vi "Lab Panel V4.91.vi"() -> ()   [LabVIEW 2013] (continued)
                          tunnel: w4008 -> [_ _]
                          tunnel: w4007 -> [_ w4049]
                          tunnel: w4006 -> [_ w4048]
                          tunnel: w4005 -> [_ w4013]
                          tunnel: w4002 -> [_ w4045]
                          tunnel: w4001 -> [_ w4044]
                          tunnel: w4000 -> [_ w4042]
                          tunnel: w3999 -> [_ w4034]
                          frame False {
                          }
                          frame True {
                            n2185 = local read "TDMS LAB02-2"() -> (w4047:refnum<k34>)
                            n2186 = Build Array(w4044) -> (w4039:dbl[])
                            n2187 = Build Array(w4042) -> (w4038:dbl[])
                            n2188 = Build Array(w4049) -> (w4037:dbl[])
                            n2189 = Build Array(w4050) -> (w4036:dbl[])
                            n2190 = Build Array(w4045) -> (w4041:dbl[])
                            n2191 = Build Array(w4043) -> (w4040:dbl[])
                            n2192 = Build Array(w4048) -> (w4035:dbl[])
                            n2193 = Build Array("AMPS ON", "AMPS OFF", "VOLTS", "PF", "TEMP Live", "TEMP Neut", "CYCLE") -> (w4018:string[])
                            n2194 = Bundle By Name("Y"=w4041, "t0"=w4034) -> (w4033:waveform(dbl))  [unwired: 1 in]
                            n2195 = Bundle By Name("Y"=w4040, "t0"=w4034) -> (w4032:waveform(dbl))  [unwired: 1 in]
                            n2196 = Bundle By Name("Y"=w4039, "t0"=w4034) -> (w4031:waveform(dbl))  [unwired: 1 in]
                            n2197 = Bundle By Name("Y"=w4038, "t0"=w4034) -> (w4030:waveform(dbl))  [unwired: 1 in]
                            n2198 = Bundle By Name("Y"=w4037, "t0"=w4034) -> (w4029:waveform(dbl))  [unwired: 1 in]
                            n2199 = Bundle By Name("Y"=w4036, "t0"=w4034) -> (w4028:waveform(dbl))  [unwired: 1 in]
                            n2200 = Bundle By Name("Y"=w4035, "t0"=w4034) -> (w4027:waveform(dbl))  [unwired: 1 in]
                            n2201 = Build Array(w4033, w4032, w4031, w4030, w4029, w4028, w4027) -> (w4026:waveform(dbl)[])
                            n2202 = TDMS Write(0:w4047, 5:"TEST VALUES", 7:w4018, 9:w4026) -> (4:w4017:refnum<k34>, 6:w4016:string, 15:w4015:errorcluster)  [unwired: 2 in, 1 out]
                            n2203 = TDMS Write(0:w4017, 5:w4016, 7:"TIME", 9:w4013, 11:w4015) -> (15:w4012:errorcluster)  [unwired: 1 in, 3 out]
                            n2204 = local write "data file error"(w4012) -> ()
                          }
                        }
                      }
                    }
                  }
                }
              }
              frame #4 {
                n2205 = case shown="True" w4051 {
                  tunnel: w4055 -> [_ w4060]
                  tunnel: w4054 -> [_ w4059]
                  tunnel: w4053 -> [_ w4057]
                  tunnel: w4052 -> [_ w4056]
                  frame False {
                  }
                  frame True {
                    n2206 = local read "DISP LAB03-1"() -> (w4061:T4)
                    n2207 = local read "SIG LAB03-1"() -> (w4062:T2)
                    n2208 = local read "ON L03-1"() -> (w4058:cluster{"amps":dbl, "volts":dbl, "pf":dbl})
                    n2209 = Unbundle(w4062) -> ("AMPS"=w4068:dbl, "VOLTS"=w4066:dbl, "PF"=w4065:dbl, "Tmp Live"=w4064:dbl, "Tmp Neut"=w4067:dbl)
                    n2210 = Unbundle(w4061) -> ("CYCLE"=w4063:dbl)  [unwired: 2 out]
                    n2211 = stacked-sequence {
                      tunnel: w4068 -> [w4072 w4091]
                      tunnel: w4067 -> [_ w4090]
                      tunnel: w4066 -> [w4071 w4089]
                      tunnel: w4065 -> [w4070 w4088]
                      tunnel: w4064 -> [_ w4087]
                      tunnel: w4063 -> [_ w4086]
                      tunnel: w4060 -> [_ w4085]
                      tunnel: w4059 -> [w4073 _]
                      tunnel: w4058 -> [w4069 w4083]
                      tunnel: w4057 -> [_ w4084]
                      tunnel: w4056 -> [_ w4079]
                      frame #0 {
                        n2212 = case shown="True" w4073 {
                          tunnel: w4072 -> [_ w4078]
                          tunnel: w4071 -> [_ w4077]
                          tunnel: w4070 -> [_ w4076]
                          tunnel: w4069 -> [_ w4074]
                          frame False {
                          }
                          frame True {
                            n2213 = Bundle(cluster=w4074, "amps"=w4078, "volts"=w4077, "pf"=w4076) -> (w4075:cluster{"amps":dbl, "volts":dbl, "pf":dbl})
                            n2214 = local write "ON L03-1"(w4075) -> ()
                          }
                        }
                      }
                      frame #1 {
                        n2215 = Unbundle(w4083) -> ("amps"=w4082:dbl, "volts"=w4081:dbl, "pf"=w4080:dbl)
                        n2216 = case shown="True" w4084 {
                          tunnel: w4091 -> [_ w4123]
                          tunnel: w4090 -> [_ w4130]
                          tunnel: w4089 -> [_ _]
                          tunnel: w4088 -> [_ _]
                          tunnel: w4087 -> [_ w4129]
                          tunnel: w4086 -> [_ w4128]
                          tunnel: w4085 -> [_ w4093]
                          tunnel: w4082 -> [_ w4125]
                          tunnel: w4081 -> [_ w4124]
                          tunnel: w4080 -> [_ w4122]
                          tunnel: w4079 -> [_ w4114]
                          frame False {
                          }
                          frame True {
                            n2217 = local read "TDMS LAB03-1"() -> (w4127:refnum<k34>)
                            n2218 = Build Array(w4124) -> (w4119:dbl[])
                            n2219 = Build Array(w4122) -> (w4118:dbl[])
                            n2220 = Build Array(w4129) -> (w4117:dbl[])
                            n2221 = Build Array(w4130) -> (w4116:dbl[])
                            n2222 = Build Array(w4125) -> (w4121:dbl[])
                            n2223 = Build Array(w4123) -> (w4120:dbl[])
                            n2224 = Build Array(w4128) -> (w4115:dbl[])
                            n2225 = Build Array("AMPS ON", "AMPS OFF", "VOLTS", "PF", "TEMP Live", "TEMP Neut", "CYCLE") -> (w4098:string[])
                            n2226 = Bundle By Name("Y"=w4121, "t0"=w4114) -> (w4113:waveform(dbl))  [unwired: 1 in]
                            n2227 = Bundle By Name("Y"=w4120, "t0"=w4114) -> (w4112:waveform(dbl))  [unwired: 1 in]
                            n2228 = Bundle By Name("Y"=w4119, "t0"=w4114) -> (w4111:waveform(dbl))  [unwired: 1 in]
                            n2229 = Bundle By Name("Y"=w4118, "t0"=w4114) -> (w4110:waveform(dbl))  [unwired: 1 in]
                            n2230 = Bundle By Name("Y"=w4117, "t0"=w4114) -> (w4109:waveform(dbl))  [unwired: 1 in]
                            n2231 = Bundle By Name("Y"=w4116, "t0"=w4114) -> (w4108:waveform(dbl))  [unwired: 1 in]
                            n2232 = Bundle By Name("Y"=w4115, "t0"=w4114) -> (w4107:waveform(dbl))  [unwired: 1 in]
                            n2233 = Build Array(w4113, w4112, w4111, w4110, w4109, w4108, w4107) -> (w4106:waveform(dbl)[])
                            n2234 = TDMS Write(0:w4127, 5:"TEST VALUES", 7:w4098, 9:w4106) -> (4:w4097:refnum<k34>, 6:w4096:string, 15:w4095:errorcluster)  [unwired: 2 in, 1 out]
                            n2235 = TDMS Write(0:w4097, 5:w4096, 7:"TIME", 9:w4093, 11:w4095) -> (15:w4092:errorcluster)  [unwired: 1 in, 3 out]
                            n2236 = local write "data file error"(w4092) -> ()
                          }
                        }
                      }
                    }
                  }
                }
              }
              frame #5 {
                n2237 = case shown="True" w4131 {
                  tunnel: w4135 -> [_ w4140]
                  tunnel: w4134 -> [_ w4139]
                  tunnel: w4133 -> [_ w4137]
                  tunnel: w4132 -> [_ w4136]
                  frame False {
                  }
                  frame True {
                    n2238 = local read "DISP LAB03-2"() -> (w4141:T4)
                    n2239 = local read "SIG LAB03-2"() -> (w4142:T2)
                    n2240 = local read "ON L03-2"() -> (w4138:cluster{"amps":dbl, "volts":dbl, "pf":dbl})
                    n2241 = Unbundle(w4142) -> ("AMPS"=w4148:dbl, "VOLTS"=w4146:dbl, "PF"=w4145:dbl, "Tmp Live"=w4144:dbl, "Tmp Neut"=w4147:dbl)
                    n2242 = Unbundle(w4141) -> ("CYCLE"=w4143:dbl)  [unwired: 2 out]
                    n2243 = stacked-sequence {
                      tunnel: w4148 -> [w4152 w4171]
                      tunnel: w4147 -> [_ w4170]
                      tunnel: w4146 -> [w4151 w4169]
                      tunnel: w4145 -> [w4150 w4168]
                      tunnel: w4144 -> [_ w4167]
                      tunnel: w4143 -> [_ w4166]
                      tunnel: w4140 -> [_ w4165]
                      tunnel: w4139 -> [w4153 _]
                      tunnel: w4138 -> [w4149 w4163]
                      tunnel: w4137 -> [_ w4164]
                      tunnel: w4136 -> [_ w4159]
                      frame #0 {
                        n2244 = case shown="True" w4153 {
                          tunnel: w4152 -> [_ w4158]
                          tunnel: w4151 -> [_ w4157]
                          tunnel: w4150 -> [_ w4156]
                          tunnel: w4149 -> [_ w4154]
                          frame False {
                          }
                          frame True {
                            n2245 = Bundle(cluster=w4154, "amps"=w4158, "volts"=w4157, "pf"=w4156) -> (w4155:cluster{"amps":dbl, "volts":dbl, "pf":dbl})
                            n2246 = local write "ON L03-2"(w4155) -> ()
                          }
                        }
                      }
                      frame #1 {
                        n2247 = Unbundle(w4163) -> ("amps"=w4162:dbl, "volts"=w4161:dbl, "pf"=w4160:dbl)
                        n2248 = case shown="True" w4164 {
                          tunnel: w4171 -> [_ w4203]
                          tunnel: w4170 -> [_ w4210]
                          tunnel: w4169 -> [_ _]
                          tunnel: w4168 -> [_ _]
                          tunnel: w4167 -> [_ w4209]
                          tunnel: w4166 -> [_ w4208]
                          tunnel: w4165 -> [_ w4173]
                          tunnel: w4162 -> [_ w4205]
                          tunnel: w4161 -> [_ w4204]
                          tunnel: w4160 -> [_ w4202]
                          tunnel: w4159 -> [_ w4194]
                          frame False {
                          }
                          frame True {
                            n2249 = local read "TDMS LAB03-2"() -> (w4207:refnum<k34>)
                            n2250 = Build Array(w4204) -> (w4199:dbl[])
                            n2251 = Build Array(w4202) -> (w4198:dbl[])
                            n2252 = Build Array(w4209) -> (w4197:dbl[])
                            n2253 = Build Array(w4210) -> (w4196:dbl[])
                            n2254 = Build Array(w4205) -> (w4201:dbl[])
                            n2255 = Build Array(w4203) -> (w4200:dbl[])
                            n2256 = Build Array(w4208) -> (w4195:dbl[])
                            n2257 = Build Array("AMPS ON", "AMPS OFF", "VOLTS", "PF", "TEMP Live", "TEMP Neut", "CYCLE") -> (w4178:string[])
                            n2258 = Bundle By Name("Y"=w4201, "t0"=w4194) -> (w4193:waveform(dbl))  [unwired: 1 in]
                            n2259 = Bundle By Name("Y"=w4200, "t0"=w4194) -> (w4192:waveform(dbl))  [unwired: 1 in]
                            n2260 = Bundle By Name("Y"=w4199, "t0"=w4194) -> (w4191:waveform(dbl))  [unwired: 1 in]
                            n2261 = Bundle By Name("Y"=w4198, "t0"=w4194) -> (w4190:waveform(dbl))  [unwired: 1 in]
                            n2262 = Bundle By Name("Y"=w4197, "t0"=w4194) -> (w4189:waveform(dbl))  [unwired: 1 in]
                            n2263 = Bundle By Name("Y"=w4196, "t0"=w4194) -> (w4188:waveform(dbl))  [unwired: 1 in]
                            n2264 = Bundle By Name("Y"=w4195, "t0"=w4194) -> (w4187:waveform(dbl))  [unwired: 1 in]
                            n2265 = Build Array(w4193, w4192, w4191, w4190, w4189, w4188, w4187) -> (w4186:waveform(dbl)[])
                            n2266 = TDMS Write(0:w4207, 5:"TEST VALUES", 7:w4178, 9:w4186) -> (4:w4177:refnum<k34>, 6:w4176:string, 15:w4175:errorcluster)  [unwired: 2 in, 1 out]
                            n2267 = TDMS Write(0:w4177, 5:w4176, 7:"TIME", 9:w4173, 11:w4175) -> (15:w4172:errorcluster)  [unwired: 1 in, 3 out]
                            n2268 = local write "data file error"(w4172) -> ()
                          }
                        }
                      }
                    }
                  }
                }
              }
              frame #6 {
                n2269 = case shown="True" w4211 {
                  tunnel: w4215 -> [_ w4220]
                  tunnel: w4214 -> [_ w4219]
                  tunnel: w4213 -> [_ w4217]
                  tunnel: w4212 -> [_ w4216]
                  frame False {
                  }
                  frame True {
                    n2270 = local read "DISP LAB04-1"() -> (w4221:T4)
                    n2271 = local read "SIG LAB04-1"() -> (w4222:T2)
                    n2272 = local read "ON L04-1"() -> (w4218:cluster{"amps":dbl, "volts":dbl, "pf":dbl})
                    n2273 = Unbundle(w4222) -> ("AMPS"=w4228:dbl, "VOLTS"=w4226:dbl, "PF"=w4225:dbl, "Tmp Live"=w4224:dbl, "Tmp Neut"=w4227:dbl)
                    n2274 = Unbundle(w4221) -> ("CYCLE"=w4223:dbl)  [unwired: 2 out]
                    n2275 = stacked-sequence {
                      tunnel: w4228 -> [w4232 w4251]
                      tunnel: w4227 -> [_ w4250]
                      tunnel: w4226 -> [w4231 w4249]
                      tunnel: w4225 -> [w4230 w4248]
                      tunnel: w4224 -> [_ w4247]
                      tunnel: w4223 -> [_ w4246]
                      tunnel: w4220 -> [_ w4245]
                      tunnel: w4219 -> [w4233 _]
                      tunnel: w4218 -> [w4229 w4243]
                      tunnel: w4217 -> [_ w4244]
                      tunnel: w4216 -> [_ w4239]
                      frame #0 {
                        n2276 = case shown="True" w4233 {
                          tunnel: w4232 -> [_ w4238]
                          tunnel: w4231 -> [_ w4237]
                          tunnel: w4230 -> [_ w4236]
                          tunnel: w4229 -> [_ w4234]
                          frame False {
                          }
                          frame True {
                            n2277 = Bundle(cluster=w4234, "amps"=w4238, "volts"=w4237, "pf"=w4236) -> (w4235:cluster{"amps":dbl, "volts":dbl, "pf":dbl})
                            n2278 = local write "ON L04-1"(w4235) -> ()
                          }
                        }
                      }
                      frame #1 {
                        n2279 = Unbundle(w4243) -> ("amps"=w4242:dbl, "volts"=w4241:dbl, "pf"=w4240:dbl)
                        n2280 = case shown="True" w4244 {
                          tunnel: w4251 -> [_ w4283]
                          tunnel: w4250 -> [_ w4290]
                          tunnel: w4249 -> [_ _]
                          tunnel: w4248 -> [_ _]
                          tunnel: w4247 -> [_ w4289]
                          tunnel: w4246 -> [_ w4288]
                          tunnel: w4245 -> [_ w4253]
                          tunnel: w4242 -> [_ w4285]
                          tunnel: w4241 -> [_ w4284]
                          tunnel: w4240 -> [_ w4282]
                          tunnel: w4239 -> [_ w4274]
                          frame False {
                          }
                          frame True {
                            n2281 = local read "TDMS LAB04-1"() -> (w4287:refnum<k34>)
                            n2282 = Build Array(w4284) -> (w4279:dbl[])
                            n2283 = Build Array(w4282) -> (w4278:dbl[])
                            n2284 = Build Array(w4289) -> (w4277:dbl[])
                            n2285 = Build Array(w4290) -> (w4276:dbl[])
                            n2286 = Build Array(w4285) -> (w4281:dbl[])
                            n2287 = Build Array(w4283) -> (w4280:dbl[])
                            n2288 = Build Array(w4288) -> (w4275:dbl[])
                            n2289 = Build Array("AMPS ON", "AMPS OFF", "VOLTS", "PF", "TEMP Live", "TEMP Neut", "CYCLE") -> (w4258:string[])
                            n2290 = Bundle By Name("Y"=w4281, "t0"=w4274) -> (w4273:waveform(dbl))  [unwired: 1 in]
                            n2291 = Bundle By Name("Y"=w4280, "t0"=w4274) -> (w4272:waveform(dbl))  [unwired: 1 in]
                            n2292 = Bundle By Name("Y"=w4279, "t0"=w4274) -> (w4271:waveform(dbl))  [unwired: 1 in]
                            n2293 = Bundle By Name("Y"=w4278, "t0"=w4274) -> (w4270:waveform(dbl))  [unwired: 1 in]
                            n2294 = Bundle By Name("Y"=w4277, "t0"=w4274) -> (w4269:waveform(dbl))  [unwired: 1 in]
                            n2295 = Bundle By Name("Y"=w4276, "t0"=w4274) -> (w4268:waveform(dbl))  [unwired: 1 in]
                            n2296 = Bundle By Name("Y"=w4275, "t0"=w4274) -> (w4267:waveform(dbl))  [unwired: 1 in]
                            n2297 = Build Array(w4273, w4272, w4271, w4270, w4269, w4268, w4267) -> (w4266:waveform(dbl)[])
                            n2298 = TDMS Write(0:w4287, 5:"TEST VALUES", 7:w4258, 9:w4266) -> (4:w4257:refnum<k34>, 6:w4256:string, 15:w4255:errorcluster)  [unwired: 2 in, 1 out]
                            n2299 = TDMS Write(0:w4257, 5:w4256, 7:"TIME", 9:w4253, 11:w4255) -> (15:w4252:errorcluster)  [unwired: 1 in, 3 out]
                            n2300 = local write "data file error"(w4252) -> ()
                          }
                        }
                      }
                    }
                  }
                }
              }
              frame #7 {
                n2301 = case shown="True" w4291 {
                  tunnel: w4295 -> [_ w4300]
                  tunnel: w4294 -> [_ w4299]
                  tunnel: w4293 -> [_ w4297]
                  tunnel: w4292 -> [_ w4296]
                  frame False {
                  }
                  frame True {
                    n2302 = local read "DISP LAB04-2"() -> (w4301:T4)
                    n2303 = local read "SIG LAB04-2"() -> (w4302:T2)
                    n2304 = local read "ON L04-2"() -> (w4298:cluster{"amps":dbl, "volts":dbl, "pf":dbl})
                    n2305 = Unbundle(w4302) -> ("AMPS"=w4308:dbl, "VOLTS"=w4306:dbl, "PF"=w4305:dbl, "Tmp Live"=w4304:dbl, "Tmp Neut"=w4307:dbl)
                    n2306 = Unbundle(w4301) -> ("CYCLE"=w4303:dbl)  [unwired: 2 out]
                    n2307 = stacked-sequence {
                      tunnel: w4308 -> [w4312 w4331]
                      tunnel: w4307 -> [_ w4330]
                      tunnel: w4306 -> [w4311 w4329]
                      tunnel: w4305 -> [w4310 w4328]
                      tunnel: w4304 -> [_ w4327]
                      tunnel: w4303 -> [_ w4326]
                      tunnel: w4300 -> [_ w4325]
                      tunnel: w4299 -> [w4313 _]
                      tunnel: w4298 -> [w4309 w4323]
                      tunnel: w4297 -> [_ w4324]
                      tunnel: w4296 -> [_ w4319]
                      frame #0 {
                        n2308 = case shown="True" w4313 {
                          tunnel: w4312 -> [_ w4318]
                          tunnel: w4311 -> [_ w4317]
                          tunnel: w4310 -> [_ w4316]
                          tunnel: w4309 -> [_ w4314]
                          frame False {
                          }
                          frame True {
                            n2309 = Bundle(cluster=w4314, "amps"=w4318, "volts"=w4317, "pf"=w4316) -> (w4315:cluster{"amps":dbl, "volts":dbl, "pf":dbl})
                            n2310 = local write "ON L04-2"(w4315) -> ()
                          }
                        }
                      }
                      frame #1 {
                        n2311 = Unbundle(w4323) -> ("amps"=w4322:dbl, "volts"=w4321:dbl, "pf"=w4320:dbl)
                        n2312 = case shown="True" w4324 {
                          tunnel: w4331 -> [_ w4363]
                          tunnel: w4330 -> [_ w4370]
                          tunnel: w4329 -> [_ _]
                          tunnel: w4328 -> [_ _]
                          tunnel: w4327 -> [_ w4369]
                          tunnel: w4326 -> [_ w4368]
                          tunnel: w4325 -> [_ w4333]
                          tunnel: w4322 -> [_ w4365]
                          tunnel: w4321 -> [_ w4364]
                          tunnel: w4320 -> [_ w4362]
                          tunnel: w4319 -> [_ w4354]
                          frame False {
                          }
                          frame True {
                            n2313 = local read "TDMS LAB04-2"() -> (w4367:refnum<k34>)
                            n2314 = Build Array(w4364) -> (w4359:dbl[])
                            n2315 = Build Array(w4362) -> (w4358:dbl[])
                            n2316 = Build Array(w4369) -> (w4357:dbl[])
                            n2317 = Build Array(w4370) -> (w4356:dbl[])
                            n2318 = Build Array(w4365) -> (w4361:dbl[])
                            n2319 = Build Array(w4363) -> (w4360:dbl[])
                            n2320 = Build Array(w4368) -> (w4355:dbl[])
                            n2321 = Build Array("AMPS ON", "AMPS OFF", "VOLTS", "PF", "TEMP Live", "TEMP Neut", "CYCLE") -> (w4338:string[])
                            n2322 = Bundle By Name("Y"=w4361, "t0"=w4354) -> (w4353:waveform(dbl))  [unwired: 1 in]
                            n2323 = Bundle By Name("Y"=w4360, "t0"=w4354) -> (w4352:waveform(dbl))  [unwired: 1 in]
                            n2324 = Bundle By Name("Y"=w4359, "t0"=w4354) -> (w4351:waveform(dbl))  [unwired: 1 in]
                            n2325 = Bundle By Name("Y"=w4358, "t0"=w4354) -> (w4350:waveform(dbl))  [unwired: 1 in]
                            n2326 = Bundle By Name("Y"=w4357, "t0"=w4354) -> (w4349:waveform(dbl))  [unwired: 1 in]
                            n2327 = Bundle By Name("Y"=w4356, "t0"=w4354) -> (w4348:waveform(dbl))  [unwired: 1 in]
                            n2328 = Bundle By Name("Y"=w4355, "t0"=w4354) -> (w4347:waveform(dbl))  [unwired: 1 in]
                            n2329 = Build Array(w4353, w4352, w4351, w4350, w4349, w4348, w4347) -> (w4346:waveform(dbl)[])
                            n2330 = TDMS Write(0:w4367, 5:"TEST VALUES", 7:w4338, 9:w4346) -> (4:w4337:refnum<k34>, 6:w4336:string, 15:w4335:errorcluster)  [unwired: 2 in, 1 out]
                            n2331 = TDMS Write(0:w4337, 5:w4336, 7:"TIME", 9:w4333, 11:w4335) -> (15:w4332:errorcluster)  [unwired: 1 in, 3 out]
                            n2332 = local write "data file error"(w4332) -> ()
                          }
                        }
                      }
                    }
                  }
                }
              }
              frame #8 {
                n2333 = case shown="True" w4371 {
                  tunnel: w4375 -> [_ w4380]
                  tunnel: w4374 -> [_ w4379]
                  tunnel: w4373 -> [_ w4377]
                  tunnel: w4372 -> [_ w4376]
                  frame False {
                  }
                  frame True {
                    n2334 = local read "DISP LAB05-1"() -> (w4381:T4)
                    n2335 = local read "SIG LAB05-1"() -> (w4382:T2)
                    n2336 = local read "ON L05-1"() -> (w4378:cluster{"amps":dbl, "volts":dbl, "pf":dbl})
                    n2337 = Unbundle(w4382) -> ("AMPS"=w4388:dbl, "VOLTS"=w4386:dbl, "PF"=w4385:dbl, "Tmp Live"=w4384:dbl, "Tmp Neut"=w4387:dbl)
                    n2338 = Unbundle(w4381) -> ("CYCLE"=w4383:dbl)  [unwired: 2 out]
                    n2339 = stacked-sequence {
                      tunnel: w4388 -> [w4392 w4411]
                      tunnel: w4387 -> [_ w4410]
                      tunnel: w4386 -> [w4391 w4409]
                      tunnel: w4385 -> [w4390 w4408]
                      tunnel: w4384 -> [_ w4407]
                      tunnel: w4383 -> [_ w4406]
                      tunnel: w4380 -> [_ w4405]
                      tunnel: w4379 -> [w4393 _]
                      tunnel: w4378 -> [w4389 w4403]
                      tunnel: w4377 -> [_ w4404]
                      tunnel: w4376 -> [_ w4399]
                      frame #0 {
                        n2340 = case shown="True" w4393 {
                          tunnel: w4392 -> [_ w4398]
                          tunnel: w4391 -> [_ w4397]
                          tunnel: w4390 -> [_ w4396]
                          tunnel: w4389 -> [_ w4394]
                          frame False {
                          }
                          frame True {
                            n2341 = Bundle(cluster=w4394, "amps"=w4398, "volts"=w4397, "pf"=w4396) -> (w4395:cluster{"amps":dbl, "volts":dbl, "pf":dbl})
                            n2342 = local write "ON L05-1"(w4395) -> ()
                          }
                        }
                      }
                      frame #1 {
                        n2343 = Unbundle(w4403) -> ("amps"=w4402:dbl, "volts"=w4401:dbl, "pf"=w4400:dbl)
                        n2344 = case shown="True" w4404 {
                          tunnel: w4411 -> [_ w4443]
                          tunnel: w4410 -> [_ w4450]
                          tunnel: w4409 -> [_ _]
                          tunnel: w4408 -> [_ _]
                          tunnel: w4407 -> [_ w4449]
                          tunnel: w4406 -> [_ w4448]
                          tunnel: w4405 -> [_ w4413]
                          tunnel: w4402 -> [_ w4445]
                          tunnel: w4401 -> [_ w4444]
                          tunnel: w4400 -> [_ w4442]
                          tunnel: w4399 -> [_ w4434]
                          frame False {
                          }
                          frame True {
                            n2345 = local read "TDMS LAB05-1"() -> (w4447:refnum<k34>)
                            n2346 = Build Array(w4444) -> (w4439:dbl[])
                            n2347 = Build Array(w4442) -> (w4438:dbl[])
                            n2348 = Build Array(w4449) -> (w4437:dbl[])
                            n2349 = Build Array(w4450) -> (w4436:dbl[])
                            n2350 = Build Array(w4445) -> (w4441:dbl[])
                            n2351 = Build Array(w4443) -> (w4440:dbl[])
                            n2352 = Build Array(w4448) -> (w4435:dbl[])
                            n2353 = Build Array("AMPS ON", "AMPS OFF", "VOLTS", "PF", "TEMP Live", "TEMP Neut", "CYCLE") -> (w4418:string[])
                            n2354 = Bundle By Name("Y"=w4441, "t0"=w4434) -> (w4433:waveform(dbl))  [unwired: 1 in]
                            n2355 = Bundle By Name("Y"=w4440, "t0"=w4434) -> (w4432:waveform(dbl))  [unwired: 1 in]
                            n2356 = Bundle By Name("Y"=w4439, "t0"=w4434) -> (w4431:waveform(dbl))  [unwired: 1 in]
                            n2357 = Bundle By Name("Y"=w4438, "t0"=w4434) -> (w4430:waveform(dbl))  [unwired: 1 in]
                            n2358 = Bundle By Name("Y"=w4437, "t0"=w4434) -> (w4429:waveform(dbl))  [unwired: 1 in]
                            n2359 = Bundle By Name("Y"=w4436, "t0"=w4434) -> (w4428:waveform(dbl))  [unwired: 1 in]
                            n2360 = Bundle By Name("Y"=w4435, "t0"=w4434) -> (w4427:waveform(dbl))  [unwired: 1 in]
                            n2361 = Build Array(w4433, w4432, w4431, w4430, w4429, w4428, w4427) -> (w4426:waveform(dbl)[])
                            n2362 = TDMS Write(0:w4447, 5:"TEST VALUES", 7:w4418, 9:w4426) -> (4:w4417:refnum<k34>, 6:w4416:string, 15:w4415:errorcluster)  [unwired: 2 in, 1 out]
                            n2363 = TDMS Write(0:w4417, 5:w4416, 7:"TIME", 9:w4413, 11:w4415) -> (15:w4412:errorcluster)  [unwired: 1 in, 3 out]
                            n2364 = local write "data file error"(w4412) -> ()
                          }
                        }
                      }
                    }
                  }
                }
              }
              frame #9 {
                n2365 = case shown="True" w4451 {
                  tunnel: w4455 -> [_ w4460]
                  tunnel: w4454 -> [_ w4459]
                  tunnel: w4453 -> [_ w4457]
                  tunnel: w4452 -> [_ w4456]
                  frame False {
                  }
                  frame True {
                    n2366 = local read "DISP LAB05-2"() -> (w4461:T4)
                    n2367 = local read "SIG LAB05-2"() -> (w4462:T2)
                    n2368 = local read "ON L05-2"() -> (w4458:cluster{"amps":dbl, "volts":dbl, "pf":dbl})
                    n2369 = Unbundle(w4462) -> ("AMPS"=w4468:dbl, "VOLTS"=w4466:dbl, "PF"=w4465:dbl, "Tmp Live"=w4464:dbl, "Tmp Neut"=w4467:dbl)
                    n2370 = Unbundle(w4461) -> ("CYCLE"=w4463:dbl)  [unwired: 2 out]
                    n2371 = stacked-sequence {
                      tunnel: w4468 -> [w4472 w4491]
                      tunnel: w4467 -> [_ w4490]
                      tunnel: w4466 -> [w4471 w4489]
                      tunnel: w4465 -> [w4470 w4488]
                      tunnel: w4464 -> [_ w4487]
                      tunnel: w4463 -> [_ w4486]
                      tunnel: w4460 -> [_ w4485]
                      tunnel: w4459 -> [w4473 _]
                      tunnel: w4458 -> [w4469 w4483]
                      tunnel: w4457 -> [_ w4484]
                      tunnel: w4456 -> [_ w4479]
                      frame #0 {
                        n2372 = case shown="True" w4473 {
                          tunnel: w4472 -> [_ w4478]
                          tunnel: w4471 -> [_ w4477]
                          tunnel: w4470 -> [_ w4476]
                          tunnel: w4469 -> [_ w4474]
                          frame False {
                          }
                          frame True {
                            n2373 = Bundle(cluster=w4474, "amps"=w4478, "volts"=w4477, "pf"=w4476) -> (w4475:cluster{"amps":dbl, "volts":dbl, "pf":dbl})
                            n2374 = local write "ON L05-2"(w4475) -> ()
                          }
                        }
                      }
                      frame #1 {
                        n2375 = Unbundle(w4483) -> ("amps"=w4482:dbl, "volts"=w4481:dbl, "pf"=w4480:dbl)
                        n2376 = case shown="True" w4484 {
                          tunnel: w4491 -> [_ w4523]
                          tunnel: w4490 -> [_ w4530]
                          tunnel: w4489 -> [_ _]
                          tunnel: w4488 -> [_ _]
                          tunnel: w4487 -> [_ w4529]
                          tunnel: w4486 -> [_ w4528]
                          tunnel: w4485 -> [_ w4493]
                          tunnel: w4482 -> [_ w4525]
                          tunnel: w4481 -> [_ w4524]
                          tunnel: w4480 -> [_ w4522]
                          tunnel: w4479 -> [_ w4514]
                          frame False {
                          }
                          frame True {
                            n2377 = local read "TDMS LAB05-2"() -> (w4527:refnum<k34>)
                            n2378 = Build Array(w4524) -> (w4519:dbl[])
                            n2379 = Build Array(w4522) -> (w4518:dbl[])
                            n2380 = Build Array(w4529) -> (w4517:dbl[])
                            n2381 = Build Array(w4530) -> (w4516:dbl[])
                            n2382 = Build Array(w4525) -> (w4521:dbl[])
                            n2383 = Build Array(w4523) -> (w4520:dbl[])
                            n2384 = Build Array(w4528) -> (w4515:dbl[])
                            n2385 = Build Array("AMPS ON", "AMPS OFF", "VOLTS", "PF", "TEMP Live", "TEMP Neut", "CYCLE") -> (w4498:string[])
                            n2386 = Bundle By Name("Y"=w4521, "t0"=w4514) -> (w4513:waveform(dbl))  [unwired: 1 in]
                            n2387 = Bundle By Name("Y"=w4520, "t0"=w4514) -> (w4512:waveform(dbl))  [unwired: 1 in]
                            n2388 = Bundle By Name("Y"=w4519, "t0"=w4514) -> (w4511:waveform(dbl))  [unwired: 1 in]
                            n2389 = Bundle By Name("Y"=w4518, "t0"=w4514) -> (w4510:waveform(dbl))  [unwired: 1 in]
                            n2390 = Bundle By Name("Y"=w4517, "t0"=w4514) -> (w4509:waveform(dbl))  [unwired: 1 in]
                            n2391 = Bundle By Name("Y"=w4516, "t0"=w4514) -> (w4508:waveform(dbl))  [unwired: 1 in]
                            n2392 = Bundle By Name("Y"=w4515, "t0"=w4514) -> (w4507:waveform(dbl))  [unwired: 1 in]
                            n2393 = Build Array(w4513, w4512, w4511, w4510, w4509, w4508, w4507) -> (w4506:waveform(dbl)[])
                            n2394 = TDMS Write(0:w4527, 5:"TEST VALUES", 7:w4498, 9:w4506) -> (4:w4497:refnum<k34>, 6:w4496:string, 15:w4495:errorcluster)  [unwired: 2 in, 1 out]
                            n2395 = TDMS Write(0:w4497, 5:w4496, 7:"TIME", 9:w4493, 11:w4495) -> (15:w4492:errorcluster)  [unwired: 1 in, 3 out]
                            n2396 = local write "data file error"(w4492) -> ()
                          }
                        }
                      }
                    }
                  }
                }
              }
            }
          }
          frame #13 {
            # "display test values on chart"
            n2397 = local read "jig cycle"() -> (w4535:dbl)
            n2398 = local read "on loops"() -> (w4537:dbl)
            n2399 = Add(x=w4537, y=2) -> (x+y=w4534:dbl)
            n2400 = Equal?(x=w4535, y=1) -> (x = y?=w4533:bool)
            n2401 = Equal?(x=w4535, y=w4534) -> (x = y?=w4532:bool)
            n2402 = Or(x=w4533, y=w4532) -> (x .or. y?=w4531:bool)
            "graph flag" <- w4531
            n2403 = global write "Global display 3.vi" "graph flag"(w4531) -> ()
            n2404 = case shown="True" w4531 {
              frame False {
              }
              frame True {
                n2405 = local read "SIG LAB05-1"() -> (w4580:T2)
                n2406 = local read "SIG LAB04-2"() -> (w4581:T2)
                n2407 = local read "SIG LAB05-2"() -> (w4579:T2)
                n2408 = local read "SIG LAB04-1"() -> (w4582:T2)
                n2409 = local read "SIG LAB03-1"() -> (w4584:T2)
                n2410 = local read "SIG LAB03-2"() -> (w4583:T2)
                n2411 = local read "SIG LAB01-1"() -> (w4588:T2)
                n2412 = local read "SIG LAB02-2"() -> (w4585:T2)
                n2413 = local read "SIG LAB02-1"() -> (w4586:T2)
                n2414 = local read "SIG LAB01-2"() -> (w4587:T2)
                n2415 = Unbundle(w4581) -> ("AMPS"=w4571:dbl, "VOLTS"=w4561:dbl, "Tmp Live"=w4551:dbl, "Tmp Neut"=w4541:dbl)  [unwired: 1 out]
                n2416 = Unbundle(w4580) -> ("AMPS"=w4570:dbl, "VOLTS"=w4560:dbl, "Tmp Live"=w4550:dbl, "Tmp Neut"=w4540:dbl)  [unwired: 1 out]
                n2417 = Unbundle(w4579) -> ("AMPS"=w4569:dbl, "VOLTS"=w4559:dbl, "Tmp Live"=w4549:dbl, "Tmp Neut"=w4539:dbl)  [unwired: 1 out]
                n2418 = Unbundle(w4582) -> ("AMPS"=w4572:dbl, "VOLTS"=w4562:dbl, "Tmp Live"=w4552:dbl, "Tmp Neut"=w4542:dbl)  [unwired: 1 out]
                n2419 = Unbundle(w4583) -> ("AMPS"=w4573:dbl, "VOLTS"=w4563:dbl, "Tmp Live"=w4553:dbl, "Tmp Neut"=w4543:dbl)  [unwired: 1 out]
                n2420 = Unbundle(w4584) -> ("AMPS"=w4574:dbl, "VOLTS"=w4564:dbl, "Tmp Live"=w4554:dbl, "Tmp Neut"=w4544:dbl)  [unwired: 1 out]
                n2421 = Unbundle(w4585) -> ("AMPS"=w4575:dbl, "VOLTS"=w4565:dbl, "Tmp Live"=w4555:dbl, "Tmp Neut"=w4545:dbl)  [unwired: 1 out]
                n2422 = Unbundle(w4586) -> ("AMPS"=w4576:dbl, "VOLTS"=w4566:dbl, "Tmp Live"=w4556:dbl, "Tmp Neut"=w4546:dbl)  [unwired: 1 out]
                n2423 = Unbundle(w4588) -> ("AMPS"=w4578:dbl, "VOLTS"=w4568:dbl, "Tmp Live"=w4558:dbl, "Tmp Neut"=w4548:dbl)  [unwired: 1 out]
                n2424 = Unbundle(w4587) -> ("AMPS"=w4577:dbl, "VOLTS"=w4567:dbl, "Tmp Live"=w4557:dbl, "Tmp Neut"=w4547:dbl)  [unwired: 1 out]
                n2425 = stacked-sequence {
                  tunnel: w4578 -> [w4620 _ _]
                  tunnel: w4577 -> [w4619 _ _]
                  tunnel: w4576 -> [w4610 _ _]
                  tunnel: w4575 -> [w4609 _ _]
                  tunnel: w4574 -> [w4599 _ _]
                  tunnel: w4573 -> [w4598 _ _]
                  tunnel: w4572 -> [_ w4643 _]
                  tunnel: w4571 -> [_ w4642 _]
                  tunnel: w4570 -> [_ w4632 _]
                  tunnel: w4569 -> [_ w4631 _]
                  tunnel: w4568 -> [w4617 _ _]
                  tunnel: w4567 -> [w4616 _ _]
                  tunnel: w4566 -> [w4607 _ _]
                  tunnel: w4565 -> [w4606 _ _]
                  tunnel: w4564 -> [w4597 _ _]
                  tunnel: w4563 -> [w4596 _ _]
                  tunnel: w4562 -> [_ w4641 _]
                  tunnel: w4561 -> [_ w4640 _]
                  tunnel: w4560 -> [_ w4630 _]
                  tunnel: w4559 -> [_ w4629 _]
                  tunnel: w4558 -> [w4614 _ _]
                  tunnel: w4557 -> [w4612 _ _]
                  tunnel: w4556 -> [w4603 _ _]
                  tunnel: w4555 -> [w4601 _ _]
                  tunnel: w4554 -> [w4595 _ _]
                  tunnel: w4553 -> [w4593 _ _]
                  tunnel: w4552 -> [_ w4639 _]
                  tunnel: w4551 -> [_ w4637 _]
                  tunnel: w4550 -> [_ w4628 _]
                  tunnel: w4549 -> [_ w4626 _]
                  tunnel: w4548 -> [w4613 _ _]
                  tunnel: w4547 -> [w4611 _ _]
                  tunnel: w4546 -> [w4602 _ _]
                  tunnel: w4545 -> [w4600 _ _]
                  tunnel: w4544 -> [w4594 _ _]
                  tunnel: w4543 -> [w4592 _ _]
                  tunnel: w4542 -> [_ w4638 _]
                  tunnel: w4541 -> [_ w4636 _]
                  tunnel: w4540 -> [_ w4627 _]
                  tunnel: w4539 -> [_ w4625 _]
                  frame #0 {
                    n2426 = Merge Signals(w4620, w4619) -> (→"LAB01 AMPS":dynamicdata)
                    n2427 = Merge Signals(w4617, w4616) -> (→"LAB01 VOLTS":dynamicdata)
                    n2428 = Merge Signals(w4597, w4596) -> (→"LAB03 VOLTS":dynamicdata)
                    n2429 = Merge Signals(w4614, w4613, w4612, w4611) -> (→"LAB01 deg C":dynamicdata)
                    n2430 = Merge Signals(w4610, w4609) -> (→"LAB02 AMPS":dynamicdata)
                    n2431 = Merge Signals(w4603, w4602, w4601, w4600) -> (→"LAB02 deg C":dynamicdata)
                    n2432 = Merge Signals(w4595, w4594, w4593, w4592) -> (→"LAB03 deg C":dynamicdata)
                    n2433 = Merge Signals(w4607, w4606) -> (→"LAB02 VOLTS":dynamicdata)
                    n2434 = Merge Signals(w4599, w4598) -> (→"LAB03 AMPS":dynamicdata)
                  }
                  frame #1 {
                    n2435 = Merge Signals(w4630, w4629) -> (→"LAB05 VOLTS":dynamicdata)
                    n2436 = Merge Signals(w4643, w4642) -> (→"LAB04 AMPS":dynamicdata)
                    n2437 = Merge Signals(w4632, w4631) -> (→"LAB05 AMPS":dynamicdata)
                    n2438 = Merge Signals(w4628, w4627, w4626, w4625) -> (→"LAB05 deg C":dynamicdata)
                    n2439 = Merge Signals(w4639, w4638, w4637, w4636) -> (→"LAB04 deg C":dynamicdata)
                    n2440 = Merge Signals(w4641, w4640) -> (→"LAB04 VOLTS":dynamicdata)
                  }
                  frame #2 {
                    n2441 = local read "LAB05 VOLTS"() -> (w4651:dynamicdata)
                    n2442 = local read "LAB04 VOLTS"() -> (w4652:dynamicdata)
                    n2443 = local read "LAB02 VOLTS"() -> (w4654:dynamicdata)
                    n2444 = local read "LAB03 VOLTS"() -> (w4653:dynamicdata)
                    n2445 = local read "LAB05 AMPS"() -> (w4657:dynamicdata)
                    n2446 = local read "LAB01 VOLTS"() -> (w4655:dynamicdata)
                    n2447 = local read "LAB04 AMPS"() -> (w4658:dynamicdata)
                    n2448 = local read "LAB03 AMPS"() -> (w4659:dynamicdata)
                    n2449 = local read "LAB03 deg C"() -> (w4647:dynamicdata)
                    n2450 = local read "LAB02 AMPS"() -> (w4660:dynamicdata)
                    n2451 = local read "LAB04 deg C"() -> (w4646:dynamicdata)
                    n2452 = local read "LAB05 deg C"() -> (w4645:dynamicdata)
                    n2453 = local read "LAB02 deg C"() -> (w4648:dynamicdata)
                    n2454 = local read "LAB01 deg C"() -> (w4649:dynamicdata)
                    n2455 = local read "LAB01 AMPS"() -> (w4661:dynamicdata)
                    n2456 = Merge Signals(w4649, w4648, w4647, w4646, w4645) -> (w4644:dynamicdata)
                    n2457 = Merge Signals(w4661, w4660, w4659, w4658, w4657) -> (w4656:dynamicdata)
                    n2458 = Merge Signals(w4655, w4654, w4653, w4652, w4651) -> (w4650:dynamicdata)
                    n2459 = global write "Global display 3.vi" "graph volts"(w4650) -> ()
                    n2460 = global write "Global display 3.vi" "graph deg C"(w4644) -> ()
                    n2461 = global write "Global display 3.vi" "graph amps"(w4656) -> ()
                  }
                }
              }
            }
          }
          frame #14 {
            # "check for amps fail"
            # "check for cycle test & temperature rise fail conditions"
            n2462 = local read "on loops"() -> (w4688:dbl)
            n2463 = local read "jig cycle"() -> (w4685:dbl)
            n2464 = local read "jig cycle"() -> (w4690:dbl)
            n2465 = Add(x=w4688, y=3.0) -> (x+y=w4686:dbl)
            n2466 = Equal?(x=w4685, y=w4686) -> (x = y?=w4681:bool)
            n2467 = local read "Fail Loops"() -> (w4662:dbl)
            n2468 = Equal?(x=w4690, y=1.0) -> (x = y?=w4683:bool)
            n2469 = global write "Global 1.vi" "fail count"(w4662) -> ()
            n2470 = stacked-sequence {
              tunnel: w4684 -> [w4693 _ _ _ _ _ _ _ _ _]
              tunnel: w4683 -> [w4694 w4714 w4734 w4754 w4774 w4794 w4814 w4834 w4854 w4874]
              tunnel: w4682 -> [w4691 _ _ _ _ _ _ _ _ _]
              tunnel: w4681 -> [w4692 w4713 w4733 w4753 w4773 w4793 w4813 w4833 w4853 w4873]
              tunnel: w4680 -> [_ w4712 _ _ _ _ _ _ _ _]
              tunnel: w4679 -> [_ w4711 _ _ _ _ _ _ _ _]
              tunnel: w4678 -> [_ _ w4732 _ _ _ _ _ _ _]
              tunnel: w4677 -> [_ _ w4731 _ _ _ _ _ _ _]
              tunnel: w4676 -> [_ _ _ w4752 _ _ _ _ _ _]
              tunnel: w4675 -> [_ _ _ w4751 _ _ _ _ _ _]
              tunnel: w4674 -> [_ _ _ _ w4772 _ _ _ _ _]
              tunnel: w4673 -> [_ _ _ _ w4771 _ _ _ _ _]
              tunnel: w4672 -> [_ _ _ _ _ w4792 _ _ _ _]
              tunnel: w4671 -> [_ _ _ _ _ w4791 _ _ _ _]
              tunnel: w4670 -> [_ _ _ _ _ _ w4812 _ _ _]
              tunnel: w4669 -> [_ _ _ _ _ _ w4811 _ _ _]
              tunnel: w4668 -> [_ _ _ _ _ _ _ w4832 _ _]
              tunnel: w4667 -> [_ _ _ _ _ _ _ w4831 _ _]
              tunnel: w4666 -> [_ _ _ _ _ _ _ _ w4852 _]
              tunnel: w4665 -> [_ _ _ _ _ _ _ _ w4851 _]
              tunnel: w4664 -> [_ _ _ _ _ _ _ _ _ w4872]
              tunnel: w4663 -> [_ _ _ _ _ _ _ _ _ w4871]
              frame #0 {
                # "LAB01-1"
                n2471 = case shown="True" w4691 {
                  tunnel: w4694 -> [_ w4707]
                  tunnel: w4693 -> [_ w4704]
                  tunnel: w4692 -> [_ w4703]
                  frame False {
                  }
                  frame True {
                    n2472 = local read "TEMP START LAB01-1"() -> (w4709:cluster{"TL":dbl, "TN":dbl})
                    n2473 = local read "RESULT LAB01-1"() -> (w4698:bool)
                    n2474 = local read "FAIL LAB01-1"() -> (w4701:cluster{"LO":dbl, "HI":dbl})
                    n2475 = local read "TDMS LAB01-1"() -> (w4708:refnum<k34>)
                    n2476 = local read "SET LAB01-1"() -> (w4705:T5)
                    n2477 = local read "DISP LAB01-1"() -> (w4706:T4)
                    n2478 = local read "SIG LAB01-1"() -> (w4710:T2)
                    n2479 = Bundle("FAIL LAB01-1"=w4701, "SIG LAB01-1"=w4710, "TEMP START LAB01-1"=w4709, "DISP LAB01-1"=w4706, "SET LAB01-1"=w4705, "TDMS LAB01-1"=w4708) -> (w4695:T32)  [unwired: 1 in]
                    n2480 = call "sub vi - cycle&temp fail v7.vi"("Amps Lo?"=w4707, "Input Cluster"=w4695, "SELECT"=w4704, "Amps Hi?"=w4703, "Result In"=w4698) -> ("(FAIL) out"=w4700:cluster{"FAIL LO":dbl, "FAIL HI":dbl}, "(DISP) out"=w4696:T4, "T-RISE"=w4697:cluster{"T-RISE (L)":dbl, "T-RISE (N)":dbl}, "Result Out"=w4699:bool, "file error"=w4702:errorcluster)  [unwired: 10 in]
                    n2481 = local write "TEMP RISE LAB01-1"(w4697) -> ()
                    n2482 = local write "FAIL LAB01-1"(w4700) -> ()
                    n2483 = local write "DISP LAB01-1"(w4696) -> ()
                    n2484 = local write "RESULT LAB01-1"(w4699) -> ()
                    n2485 = local write "data file error"(w4702) -> ()
                  }
                }
              }
              frame #1 {
                # "LAB01-2"
                n2486 = case shown="True" w4712 {
                  tunnel: w4714 -> [_ w4727]
                  tunnel: w4711 -> [_ w4724]
                  tunnel: w4713 -> [_ w4723]
                  frame False {
                  }
                  frame True {
                    n2487 = local read "TEMP START LAB01-2"() -> (w4729:cluster{"TL":dbl, "TN":dbl})
                    n2488 = local read "FAIL LAB01-2"() -> (w4720:cluster{"LO":dbl, "HI":dbl})
                    n2489 = local read "TDMS LAB01-2"() -> (w4728:refnum<k34>)
                    n2490 = local read "SET LAB01-2"() -> (w4725:T5)
                    n2491 = local read "DISP LAB01-2"() -> (w4726:T4)
                    n2492 = local read "RESULT LAB01-2"() -> (w4717:bool)
                    n2493 = local read "SIG LAB01-2"() -> (w4730:T2)
                    n2494 = Bundle("FAIL LAB01-2"=w4720, "SIG LAB01-2"=w4730, "TEMP START LAB01-2"=w4729, "DISP LAB01-2"=w4726, "SET LAB01-2"=w4725, "TDMS LAB01-2"=w4728) -> (w4715:T33)  [unwired: 1 in]
                    n2495 = call "sub vi - cycle&temp fail v7.vi"("Amps Lo?"=w4727, "Input Cluster"=w4715, "SELECT"=w4724, "Amps Hi?"=w4723, "Result In"=w4717) -> ("(FAIL) out"=w4719:cluster{"FAIL LO":dbl, "FAIL HI":dbl}, "(DISP) out"=w4722:T4, "T-RISE"=w4716:cluster{"T-RISE (L)":dbl, "T-RISE (N)":dbl}, "Result Out"=w4718:bool, "file error"=w4721:errorcluster)  [unwired: 10 in]
                    n2496 = local write "TEMP RISE LAB01-2"(w4716) -> ()
                    n2497 = local write "FAIL LAB01-2"(w4719) -> ()
                    n2498 = local write "DISP LAB01-2"(w4722) -> ()
                    n2499 = local write "RESULT LAB01-2"(w4718) -> ()
                    n2500 = local write "data file error"(w4721) -> ()
                  }
                }
              }
              frame #2 {
                # "LAB02-1"
                n2501 = case shown="True" w4732 {
                  tunnel: w4734 -> [_ w4747]
                  tunnel: w4731 -> [_ w4744]
                  tunnel: w4733 -> [_ w4743]
                  frame False {
                  }
                  frame True {
                    n2502 = local read "TEMP START LAB02-1"() -> (w4749:cluster{"TL":dbl, "TN":dbl})
                    n2503 = local read "FAIL LAB02-1"() -> (w4740:cluster{"LO":dbl, "HI":dbl})
                    n2504 = local read "TDMS LAB02-1"() -> (w4748:refnum<k34>)
                    n2505 = local read "SET LAB02-1"() -> (w4745:T5)
                    n2506 = local read "DISP LAB02-1"() -> (w4746:T4)
                    n2507 = local read "SIG LAB02-1"() -> (w4750:T2)
                    n2508 = local read "RESULT LAB02-1"() -> (w4737:bool)
                    n2509 = Bundle("FAIL LAB02-1"=w4740, "SIG LAB02-1"=w4750, "TEMP START LAB02-1"=w4749, "DISP LAB02-1"=w4746, "SET LAB02-1"=w4745, "TDMS LAB02-1"=w4748) -> (w4735:T34)  [unwired: 1 in]
                    n2510 = call "sub vi - cycle&temp fail v7.vi"("Amps Lo?"=w4747, "Input Cluster"=w4735, "SELECT"=w4744, "Amps Hi?"=w4743, "Result In"=w4737) -> ("(FAIL) out"=w4739:cluster{"FAIL LO":dbl, "FAIL HI":dbl}, "(DISP) out"=w4742:T4, "T-RISE"=w4736:cluster{"T-RISE (L)":dbl, "T-RISE (N)":dbl}, "Result Out"=w4738:bool, "file error"=w4741:errorcluster)  [unwired: 10 in]
                    n2511 = local write "TEMP RISE LAB02-1"(w4736) -> ()
                    n2512 = local write "FAIL LAB02-1"(w4739) -> ()
                    n2513 = local write "DISP LAB02-1"(w4742) -> ()
                    n2514 = local write "RESULT LAB02-1"(w4738) -> ()
                    n2515 = local write "data file error"(w4741) -> ()
                  }
